vi "oval_plots.vi"(10 "Solution":dbl[](array[numeric]), 11 "ovalization_data":T1={"AngOval"=[0.0, 60.0, 120.0, 22.5, 45.0, 67.5, 90.0, 112.5, 135.0, 157.5, 180.0], "OvalDiam"=[324.25, 324.6, 324.55, 324.25, 324.55, 324.65, 324.6, 324.65, 324.55, 324.5, 324.4], "Plots"={"Ref"={"X"=[], "Y"=[]}, "Elipse"={"X"=[], "Y"=[]}, "Points"={"X"=[], "Y"=[]}}, "Ampliation"=100.0, "Results"={"MD"=0.0, "mD"=0.0, "Dmed"=0.0, "Oval"=0.0, "ang"=0.0, "X0"=0.0, "Y0"=0.0}}) -> (3 "output ovalization_data-out":T1={"AngOval"=[0.0, 60.0, 120.0, 22.5, 45.0, 67.5, 90.0, 112.5, 135.0, 157.5, 180.0], "OvalDiam"=[324.25, 324.6, 324.55, 324.25, 324.55, 324.65, 324.6, 324.65, 324.55, 324.5, 324.4], "Plots"={"Ref"={"X"=[], "Y"=[]}, "Elipse"={"X"=[], "Y"=[]}, "Points"={"X"=[], "Y"=[]}}, "Ampliation"=100.0, "Results"={"MD"=0.0, "mD"=0.0, "Dmed"=0.0, "Oval"=0.0, "ang"=0.0, "X0"=0.0, "Y0"=0.0}})   [LabVIEW 2016]
uses:
  ovalization_data.ctl
  <vilib>/Analysis/1siggen.llb/Ramp Pattern by Samples.vi
  <vilib>/Analysis/baseanly.llb/Mean (DBL).vi
  <vilib>/Analysis/NI_AALBase.lvlib
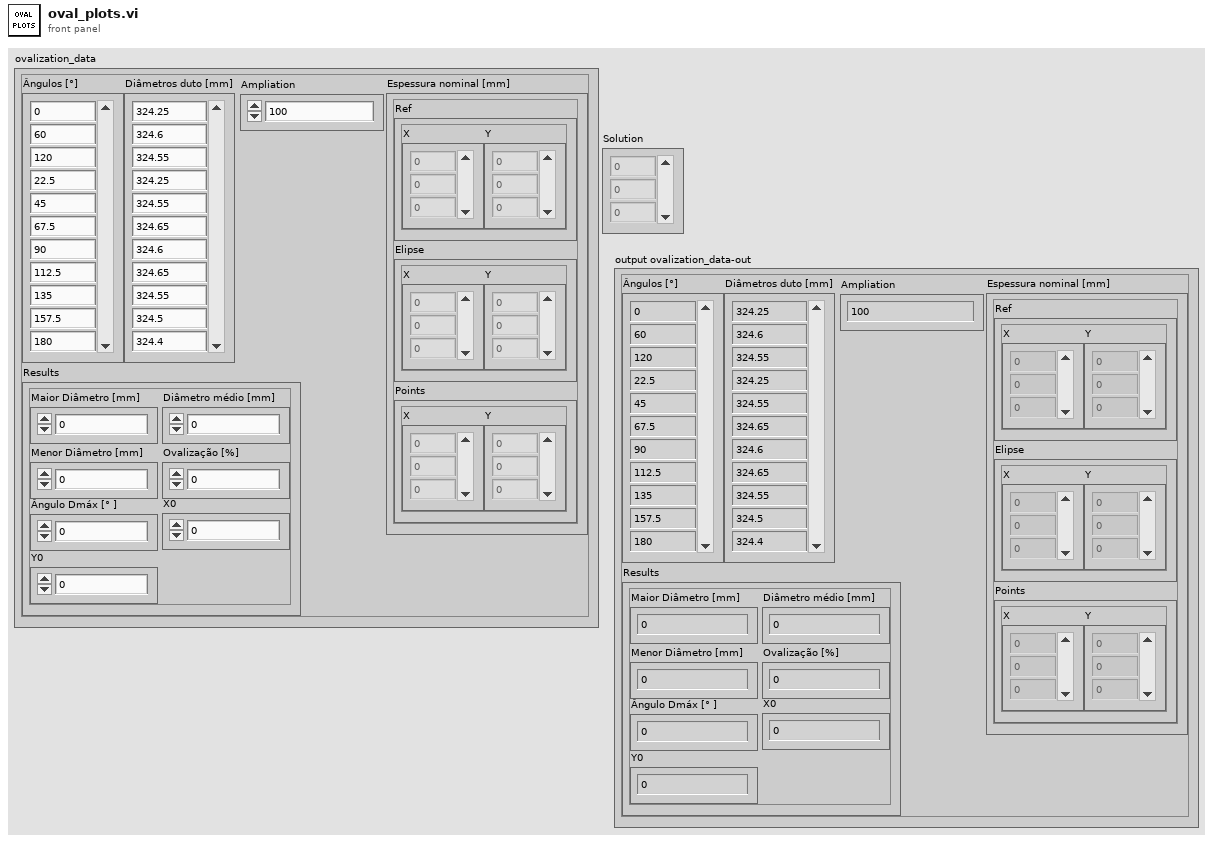
[diagram p1: front panel]
types:
  T1 = typedef "ovalization_data.ctl" = cluster{"AngOval":dbl[], "OvalDiam":dbl[], "Plots":cluster{"Ref":cluster{"X":dbl[], "Y":dbl[]}, "Elipse":cluster{"X":dbl[], "Y":dbl[]}, "Points":cluster{"X":dbl[], "Y":dbl[]}}, "Ampliation":dbl, "Results":cluster{"MD":dbl, "mD":dbl, "Dmed":dbl, "Oval":dbl, "ang":dbl, "X0":dbl, "Y0":dbl}}
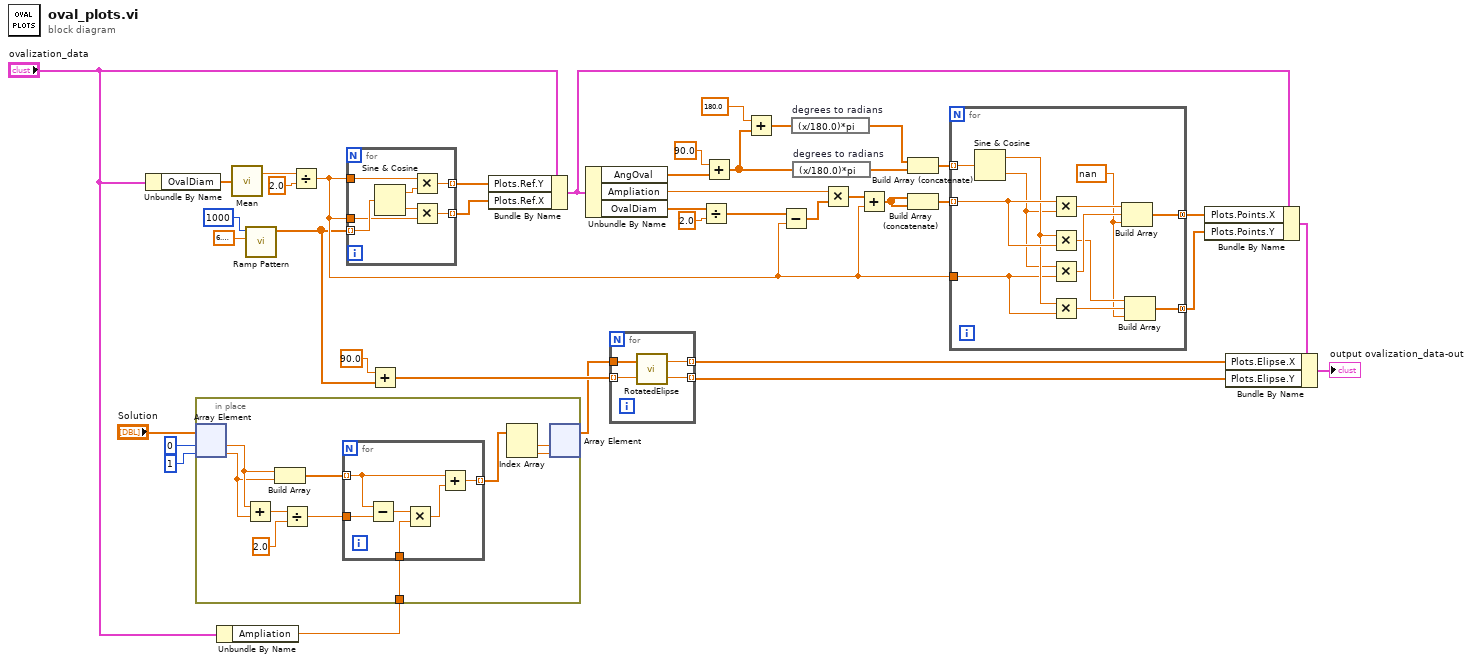
[diagram p0: block diagram]
diagram:
  n1 = Unbundle By Name("ovalization_data") -> ("OvalDiam"=w40:dbl[])
  n2 = Unbundle By Name("ovalization_data") -> ("Ampliation"=w9:dbl)
  n3 = in-place {
    in-place-border: w9 -> [w44]
    n4 = in-place-array #1("Solution", 0, 1) -> (w48:dbl, w47:dbl)
    n5 = Add(x=w48, y=w47) -> (x+y=w49:dbl)
    n6 = Build Array(w48, w47) -> (w46:dbl[])
    n7 = Divide(x=w49, y=2.0) -> (x/y=w45:dbl)
    n8 = for {
      tunnel: w46 -> [w52] mode=indexing
      tunnel: w45 -> [w56]
      tunnel: w44 -> [w54]
      tunnel: [w51] -> w43 mode=indexing
      n9 = Subtract(x=w52, y=w56) -> (x-y=w55:dbl)
      n10 = Multiply(x=w55, y=w54) -> (x*y=w53:dbl)
      n11 = Add(x=w52, y=w53) -> (x+y=w51:dbl)
    }
    n12 = Index Array(array=w43) -> (element #1=w42:dbl, element #2=w41:dbl)  [unwired: 2 in]
    n13 = in-place-array #1(w42, w41) -> (w8:dbl[])  [unwired: 2 out]
  }
  n14 = call-poly <vilib>:"Mean.vi"("X"=w40) -> ("mean"=w39:dbl)  [unwired: 1 out]
  n15 = call-poly <vilib>:"Ramp Pattern.vi"("end"=6.283185307179586, "samples"=1000) -> ("Ramp Pattern"=w13:dbl[])  [unwired: 8 in, 1 out]
  n16 = Divide(x=w39, y=2.0) -> (x/y=w26:dbl)
  n17 = for {
    tunnel: w13 -> [w63] mode=indexing
    tunnel: w26 -> [w61]
    tunnel: w26 -> [w59]
    tunnel: [w58] -> w36 mode=indexing
    tunnel: [w57] -> w35 mode=indexing
    n18 = Sine & Cosine(0:w63) -> (1:w60:dbl, 2:w62:dbl)
    n19 = Multiply(x=w59, y=w60) -> (x*y=w58:dbl)
    n20 = Multiply(x=w62, y=w61) -> (x*y=w57:dbl)
  }
  n21 = Add(x=90.0 ("y"), y=w13) -> (x+y=w12:dbl[])
  n22 = Bundle By Name(cluster="ovalization_data", "Plots.Ref.Y"=w36, "Plots.Ref.X"=w35) -> (w25:T1)
  n23 = Unbundle By Name(w25) -> ("AngOval"=w28:dbl[], "Ampliation"=w30:dbl, "OvalDiam"=w33:dbl[])
  n24 = for {
    tunnel: w12 -> [w67] mode=indexing
    tunnel: w8 -> [w66]
    tunnel: [w65] -> w3 mode=indexing
    tunnel: [w64] -> w2 mode=indexing
    n25 = call "RotatedElipse.vi"("theta"=w67, "Parameters"=w66) -> ("y out"=w64:dbl, "x out"=w65:dbl)
  }
  n26 = Divide(x=w33, y=2.0) -> (x/y=w32:dbl[])
  n27 = Add(x=90.0 ("y"), y=w28) -> (x+y=w21:dbl[])
  n28 = Add(x=180.0 ("y"), y=w21) -> (x+y=w20:dbl[])
  n29 = Subtract(x=w32, y=w26) -> (x-y=w31:dbl[])
  n30 = expression code="(x/180.0)*pi" "degrees to radians"(w20) -> (w18:dbl[])
  n31 = expression code="(x/180.0)*pi" "degrees to radians"(w21) -> (w19:dbl[])
  n32 = Multiply(x=w30, y=w31) -> (x*y=w29:dbl[])
  n33 = Add(x=w29, y=w26) -> (x+y=w16:dbl[])
  n34 = Build Array (concatenate)(w18, w19) -> (w17:dbl[])
  n35 = Build Array (concatenate)(w16, w16) -> (w15:dbl[])
  n36 = for {
    tunnel: w26 -> [w75]
    tunnel: w15 -> [w78] mode=indexing
    tunnel: w17 -> [w79] mode=indexing
    tunnel: [w69] -> w24 mode=concatenating
    tunnel: [w68] -> w23 mode=concatenating
    w70 = nan ("y")
    n37 = Sine & Cosine(0:w79) -> (1:w77:dbl, 2:w76:dbl)
    n38 = Multiply(x=w78, y=w76) -> (x*y=w74:dbl)
    n39 = Multiply(x=w77, y=w78) -> (x*y=w72:dbl)
    n40 = Multiply(x=w76, y=w75) -> (x*y=w73:dbl)
    n41 = Multiply(x=w77, y=w75) -> (x*y=w71:dbl)
    n42 = Build Array(w74, w73, w70) -> (w69:dbl[])
    n43 = Build Array(w72, w71, w70) -> (w68:dbl[])
  }
  n44 = Bundle By Name(cluster=w25, "Plots.Points.X"=w24, "Plots.Points.Y"=w23) -> (w5:T1)
  n45 = Bundle By Name(cluster=w5, "Plots.Elipse.X"=w3, "Plots.Elipse.Y"=w2) -> (→"output ovalization_data-out":T1)
